vi "database_with_data.vi"(10 "input":string) -> (0 "error":errorcluster, 2 "Data":string[][](array[string]))   [LabVIEW 2017, in "Lib_code.lvlib"]
uses:
  Lib_code.lvlib
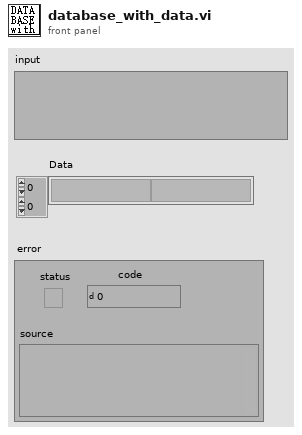
[diagram p1: front panel]
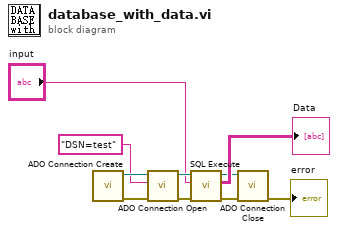
[diagram p0: block diagram]
diagram:
  n1 = call <userlib>:"ADO Connection Create.vi"() -> ("error out"=w6:errorcluster, "ADODB._Connection Out"=w3:refnum<k7>)  [unwired: 10 in]
  n2 = call <userlib>:"ADO Connection Open.vi"("error in (no error)"=w6, "ConnectionString"="DSN=test", "ADODB._Connection In"=w3) -> ("error out"=w7:errorcluster, "ADODB._Connection Out"=w4:refnum<k7>)  [unwired: 7 in]
  n3 = call <userlib>:"SQL Execute.vi"("error in (no error)"=w7, "Command Text"="input", "ADODB._Connection In"=w4) -> ("error out"=w8:errorcluster, "Data"=→"Data":string[][], "ADODB._Connection Out"=w5:refnum<k7>)  [unwired: 5 in, 1 out]
  n4 = call <userlib>:"ADO Connection Close.vi"("error in (no error)"=w8, "ADODB._Connection In"=w5) -> ("error out"=→"error":errorcluster)  [unwired: 8 in, 1 out]
